vi "DeviceSendBytesRoutedMessage_Create.vi"(7 "Header":T2, 8 "error in (no error)":errorcluster, 10 "SendTo":string, 11 "DeviceSendBytesRoutedMessage":T1) -> (0 "error out":errorcluster, 3 "Message":T4)   [LabVIEW 2017]
uses:
  <vilib>/addons/InsightCM/MessageBus/Base/controls/Message.ctl
  <vilib>/addons/InsightCM/MessageBus/Base/controls/MessageHeader.ctl
  <vilib>/addons/InsightCM/MessageBus/Base/controls/KeyValuePair.ctl
  <vilib>/addons/InsightCM/MessageBus/MessageLibrary/Device/controls/DeviceSendBytesRoutedMessageBody.ctl
  <vilib>/addons/InsightCM/MessageBus/Base/controls/MessageClassType.ctl
  <vilib>/addons/InsightCM/Utilities/PropertyHelpers/PropertyHelpers.lvlib
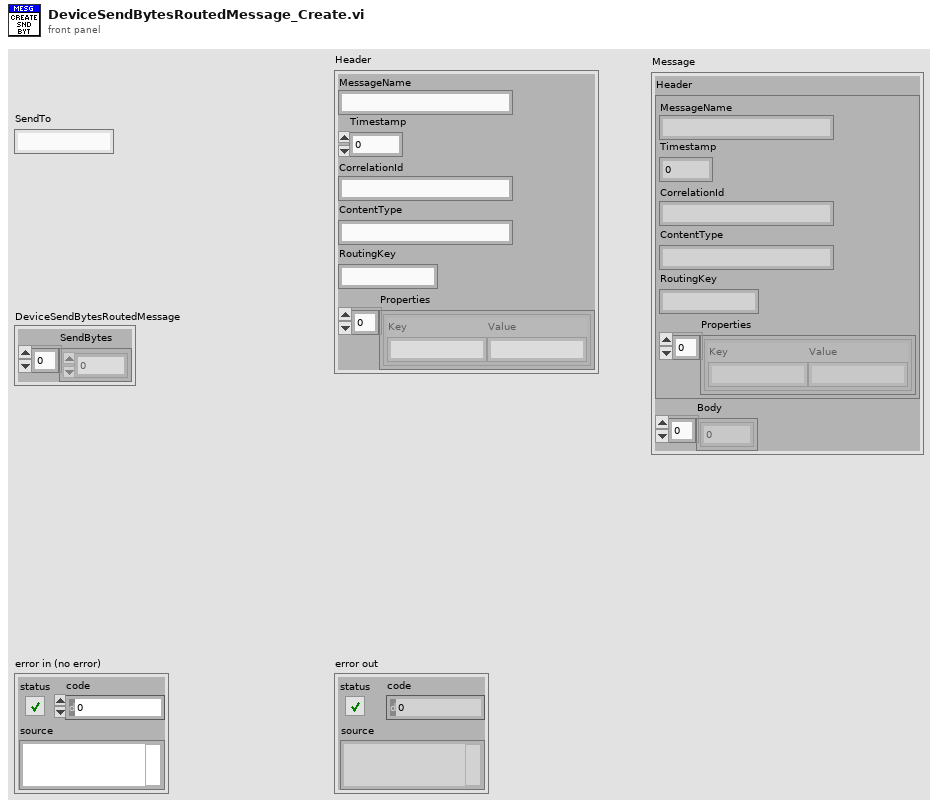
[diagram p1: front panel]
types:
  T1 = typedef "DeviceSendBytesRoutedMessageBody.ctl" = cluster{"SendBytes":u8[]}
  T2 = typedef "MessageHeader.ctl" = cluster{"MessageName":string, "Timestamp":i64, "CorrelationId":string, "ContentType":string, "RoutingKey":string, "Properties":T3[]}
  T3 = typedef "KeyValuePair.ctl" = cluster{"Key":string, "Value":string}
  T4 = typedef "Message.ctl" = cluster{"Header":T2, "Body":u8[]}
  T5 = typedef "MessageClassType.ctl" = enum16{"Request", "Response", "Broadcast", "RoutedMessage"}
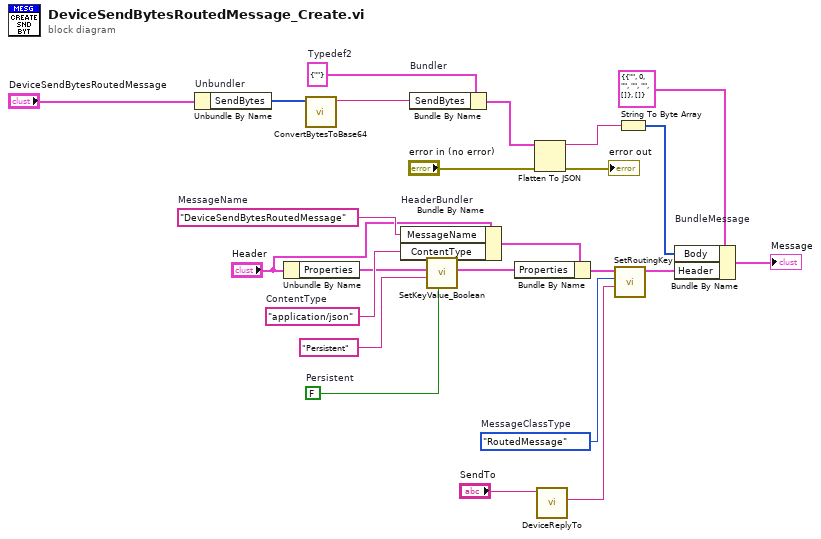
[diagram p0: block diagram]
diagram:
  w3 = cluster{"SendBytes":string} {"SendBytes"=""}  # Typedef2
  w20 = MessageClassType."RoutedMessage"  # MessageClassType
  w15 = FALSE  # Persistent
  w21 = "DeviceSendBytesRoutedMessage"  # MessageName
  w18 = "application/json"  # ContentType
  n1 = Unbundle By Name "Unbundler"("DeviceSendBytesRoutedMessage") -> ("SendBytes"=w2:u8[])
  n2 = Unbundle By Name("Header") -> ("Properties"=w17:T3[])
  n3 = call <vilib>:"ConvertBytesToBase64.vi"("U8 array"=w2) -> ("base64 encoded"=w1:string)  [unwired: 10 in]
  n4 = Bundle By Name "HeaderBundler"(cluster="Header", "MessageName"=w21, "ContentType"=w18) -> (w12:T2)
  n5 = Bundle By Name "Bundler"(cluster=w3, "SendBytes"=w1) -> (w4:cluster{"SendBytes":string})
  n6 = call <vilib>:"SetKeyValue_Boolean.vi"("value"=w15, "key"="Persistent" ("Key"), "key value pairs"=w17) -> ("key value pairs out"=w11:T3[])  [unwired: 8 in]
  n7 = Bundle By Name(cluster=w12, "Properties"=w11) -> (w13:T2)
  n8 = Flatten To JSON(anything=w4, error in (no error)="error in (no error)") -> (JSON string=w6:string, 11:→"error out":errorcluster)  [unwired: 1 in]
  n9 = call <vilib>:"DeviceReplyTo.vi"("Device"="SendTo") -> ("ReplyTo"=w7:string)  [unwired: 10 in]
  n10 = call <vilib>:"SetRoutingKey.vi"("SendTo"=w7, "MessageClassType"=w20, "Message Header in"=w13) -> ("Message Header out"=w14:T2)  [unwired: 8 in]
  n11 = String To Byte Array(string=w6) -> (unsigned byte array=w23:u8[])
  n12 = Bundle By Name "BundleMessage"(cluster=T4 {"Header"={"MessageName"="", "Timestamp"=0, "CorrelationId"="", "ContentType"="", "RoutingKey"="", "Properties"=[]}, "Body"=[]} ("Message"), "Body"=w23, "Header"=w14) -> (→"Message":T4)
